vi "CREATE DATABASE.vi"(6 "object":refnum<class "_ISerializable.lvclass">, 9 "create script 2":string, 11 "LV-ORM in":refnum<class "LV-ORM.lvclass">) -> (3 "LV-ORM out":refnum<class "LV-ORM.lvclass">)   [LabVIEW 2018, in "LV-ORM.lvclass"]
uses:
  LV-ORM.lvclass
  _Serializable Base Object/_ISerializable.lvclass
panel:
  in  "error in":errorcluster
  out "error out":errorcluster
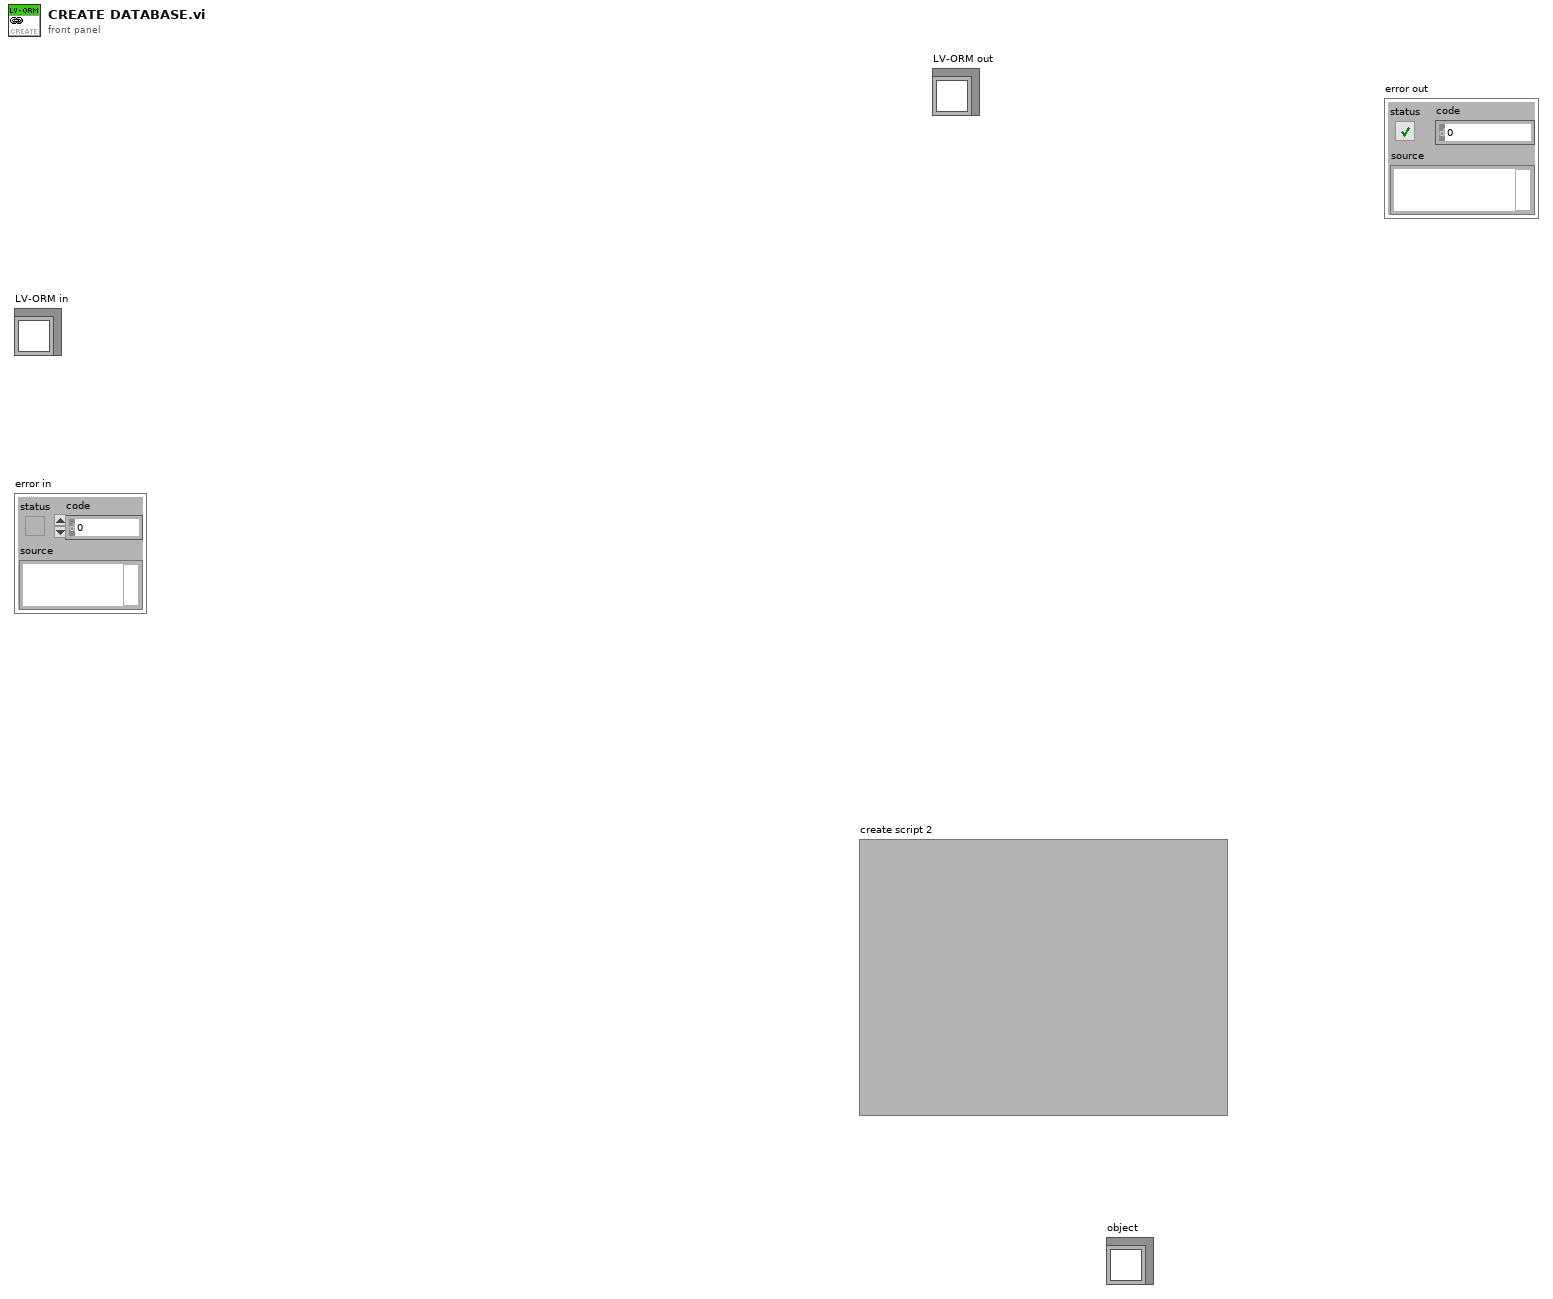
[diagram p1: front panel]
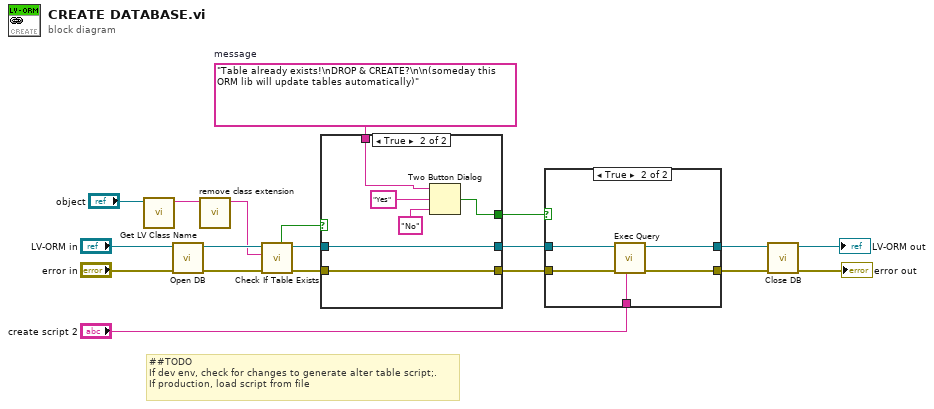
[diagram p0: block diagram]
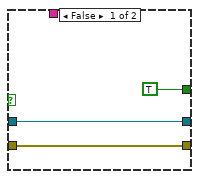
[diagram p3: hidden frame]
diagram:
  w19 = "Table already exists!\nDROP & CREATE?\n\n(someday this ORM lib will update tables automatically)"  # message
  # "##TODO\nIf dev env, check for changes to generate alter table script;.\nIf production, load script from file"
  n1 = call <vilib>:"Get LV Class Name.vi"("object"="object") -> ("class name"=w5:string)  [unwired: 9 in, 1 out]
  n2 = call "Open DB.vi"("error in (no error)"="error in", "LV-ORM in"="LV-ORM in") -> ("error out"=w13:errorcluster, "LV-ORM out"=w10:refnum<class "LV-ORM.lvclass">)  [unwired: 8 in]
  n3 = call "remove class extension.vi"("class name in"=w5) -> ("class name out"=w3:string)  [unwired: 10 in]
  n4 = call "Check If Table Exists.vi"("error in"=w13, "Table Name"=w3, "orm in"=w10) -> ("error out"=w17:errorcluster, "orm out"=w18:refnum<class "LV-ORM.lvclass">, "table exists?"=w16:bool)  [unwired: 5 in, 1 out]
  n5 = case shown="True" w16 {
    tunnel: [TRUE w23] -> w6
    tunnel: w19 -> [_ w24]
    tunnel: w18 -> [w20 w27]
    tunnel: w17 -> [w21 w28]
    tunnel: [w21 w28] -> w14
    tunnel: [w20 w27] -> w15
    frame False {
    }
    frame True {
      n6 = Two Button Dialog(message=w24, 1:"No", 2:"Yes") -> (T button?=w23:bool)
    }
  }
  n7 = case shown="True" w6 {
    tunnel: w15 -> [w30 w33]
    tunnel: w14 -> [w29 w35]
    tunnel: [w30 w32] -> w11
    tunnel: [w29 w34] -> w12
    tunnel: "create script 2" -> [_ w31]
    frame False {
    }
    frame True {
      n8 = call "Exec Query.vi"("scripts"=w31, "error in"=w35, "orm in"=w33) -> ("error out"=w34:errorcluster, "orm out"=w32:refnum<class "LV-ORM.lvclass">)  [unwired: 7 in]
    }
  }
  n9 = call "Close DB.vi"("error in"=w12, "LV-ORM in"=w11) -> ("error out"=→"error out":errorcluster, "LV-ORM out"=→"LV-ORM out":refnum<class "LV-ORM.lvclass">)  [unwired: 8 in]
